vi "Host_SetParameters.vi"() -> ()   [LabVIEW 2017]
doc: "Allows manual modification of run parameters while Host__Main.vi is running.\nParameters include: distance and time thresholds for run, direction, throttle, minimum and maximum health check values, loop periods\nVI will update all values when window is closed or when \"Close Window\" button is pressed\n\nVI is automatically called on starting Host__Main.vi in order to set loop periods in Master__Main.vi.\nIf vi is not executed before running Master__Main.vi, the cRIO will not run and will return an error."
uses:
  Master/TypeDef_RunParameters.ctl
  Master/TypeDef_LoopPeriods.ctl
  Master/DAQ/Master_DataControl.ctl
  Master/DAQ/TypeDef_cRIOData.ctl
  Master/IMU/TypeDef_IMUData.ctl
  Master/CAN/TypeDef_BMSData.ctl
  Master/CAN/TypeDef_BMS_Status.ctl
  Master/CAN/MotorController/fixedMotorData.ctl
  Master/CAN/MotorController/MotorStatus.ctl
  Globals/Host_RUNPARAMETERS.vi
panel:
  in  "Disconnect Timeout (ms)":u32=30000
  in  "driveMode":enum16{"velocityMode", "torqueMode", ""}(ring)
  in  "Service Parameters":T1={"Distance Threshold (ft)"=10000.0, "Time Threshold (s)"=10000.0, "Target (I16)"=2} {"Target (I16)" min=0 max=5 step=1}
  in  "Full Run Parameters":T1={"Distance Threshold (ft)"=2300.0, "Time Threshold (s)"=12.57, "Target (I16)"=2} {"Target (I16)" min=0 max=5 step=1}
  in  "Reinitialize Network Stream":bool
  in  "Reinitialize CAN":bool
  in  "Reset Navigation":bool
  in  "Nav Period (ms)":u32=10
  in  "Set Acceleration Offset":bool
  in  "Set Min/Max Values":string[][](table)=[["22", "29.2", "V"], ["-1", "30", "A"], ["0", "0", "V"], ["-1", "30", "psig"], ["33", "149", "°F"], ["33", "248", "°F"], ["0", "1.9", "in"], ["0", "1.9", "in"], ["250", "3000", "psig"], ["-1", "15", "psig"], ["-1", "35", "psig"], ["-2.5", "20", "psig"], ["-2", "1.5", "g"], ["0", "16", "psia"], ["-40", "185", "°F"], ["33", "175", "°F"], ["10", "91", "%"], ["0", "4.1", "V"]]
  in  "CAN Period (ms)":i64=90
  in  "IMU Period (ms)":u32=5
  in  "DAQ Period (ms)":u32=100
  in  "Control Period (ms)":i64=10
  in  "Process Stop Button":bool
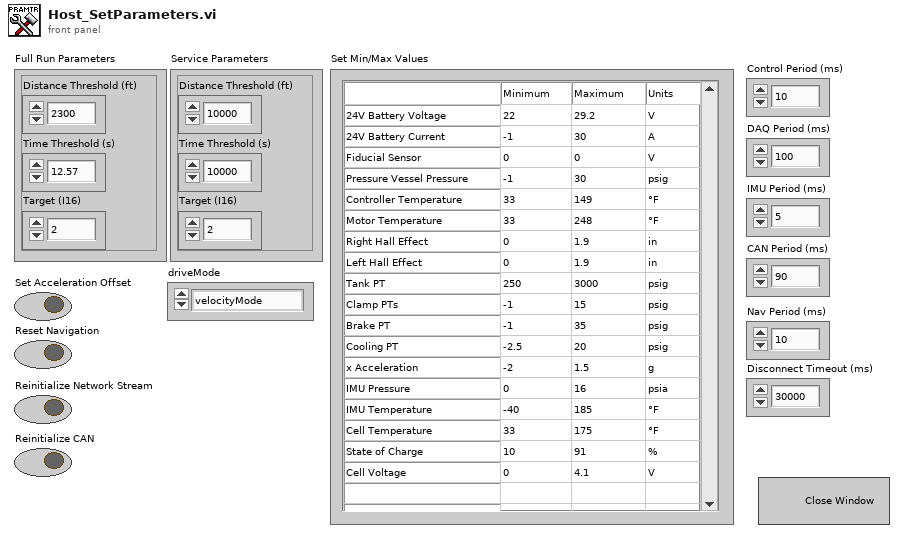
[diagram p1: front panel]
types:
  T1 = typedef "TypeDef_RunParameters.ctl" = cluster{"Distance Threshold (ft)":dbl, "Time Threshold (s)":dbl, "Target (I16)":i16}
  T2 = typedef "TypeDef_LoopPeriods.ctl" = cluster{"Control Period":i64, "DAQ Period":u32, "IMU Period":u32, "CAN Period":i64, "Nav Period":u32}
  T3 = typedef "Master_DataControl.ctl" = cluster{"cRIO Data":T4, "IMU Data":T5, "BMS Data":T6, "Motor Data":T8}
  T4 = typedef "TypeDef_cRIOData.ctl" = cluster{"Time (ms)":dbl, "24V Battery (V)":dbl, "LowV Current (A)":dbl, "Fiducial Sensor (V)":dbl, "PV Pressure (psig)":dbl, "Flow Sensor (V)":dbl, "Temp Fairing (F)":dbl, "Temp Reservoir (F)":dbl, "HallEffect Right (in)":dbl, "HallEffect Left (in)":dbl, "PT Tank (psig)":dbl, "PT Clamp Right (psig)":dbl, "PT Clamp Left (psig)":dbl, "PT Brake (psig)":dbl, "PT Cooling (psig)":dbl, "Displacement (ft)":dbl, "Velocity (ft/s)":dbl}
  T5 = typedef "TypeDef_IMUData.ctl" = cluster{"x acceleration (g)":dbl, "Pressure (psia)":dbl, "Temperature (F)":dbl}
  T6 = typedef "TypeDef_BMSData.ctl" = cluster{"Max Cell Voltage (V)":dbl, "Max Cell ID":dbl, "Min Cell Voltage (V)":dbl, "Min Cell ID":dbl, "State of Charge (%)":dbl, "Average Voltage (V)":dbl, "Voltage Delta (V)":dbl, "Pack Current (A)":dbl, "Pack Voltage (V)":dbl, "Max Resistance (Ohm)":dbl, "Min Resistance (Ohm)":dbl, "Average Resistance (Ohm)":dbl, "Delta Resistance (Ohm)":dbl, "Highest Temperature(F)":dbl, "BmsStatus":T7}
  T7 = typedef "TypeDef_BMS_Status.ctl" = cluster{"isFault":bool, "isolationMonitoring":bool}
  T8 = typedef "fixedMotorData.ctl" = cluster{"Velo (RPM)":dbl, "MotorTemp(F)":dbl, "CtrlTemp(F)":dbl, "DcLinkVolt(V)":dbl, "ErrorCode":dbl, "motorStatus":T9, "isAlive":bool, "motorControllerState":u16}
  T9 = typedef "MotorStatus.ctl" = cluster{"isReady":bool, "isOn":bool, "isOperEn":bool, "isFault":bool, "isVoltEn":bool, "targetReached":bool, "isWarning":bool}
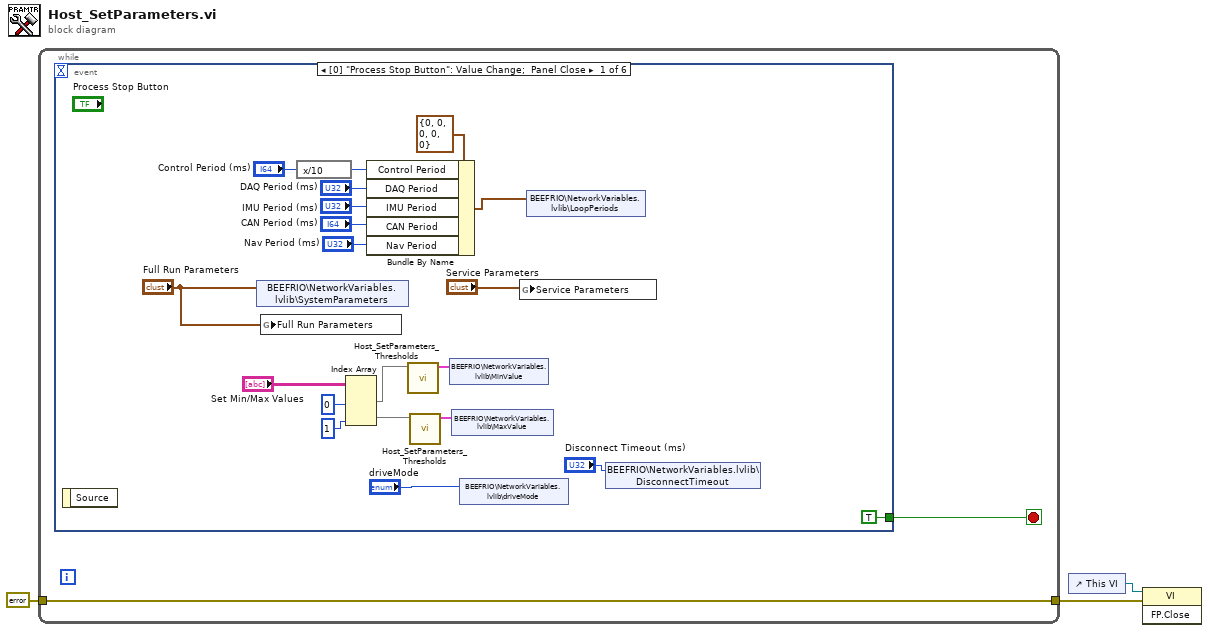
[diagram p0: block diagram]
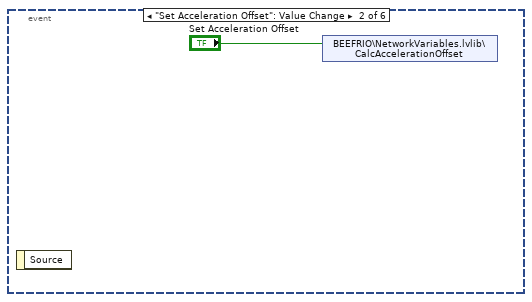
[diagram p2: hidden frame]
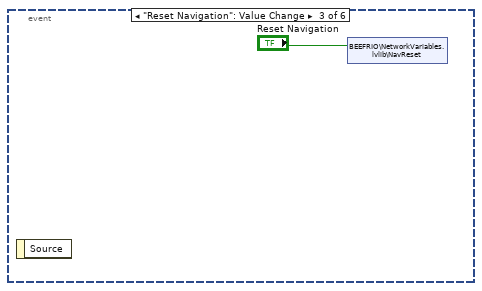
[diagram p3: hidden frame]
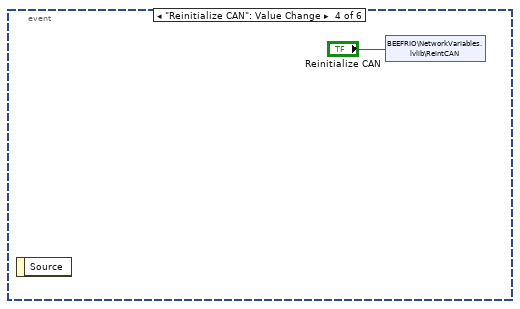
[diagram p4: hidden frame]
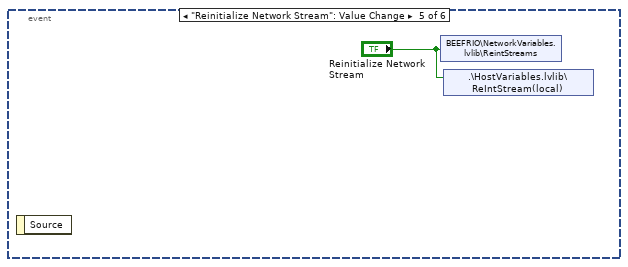
[diagram p5: hidden frame]
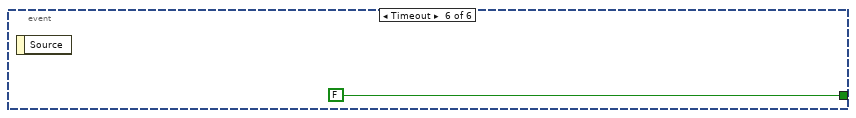
[diagram p6: hidden frame]
diagram:
  n1 = while {
    tunnel: errorcluster {"status"=FALSE, "code"=0, "source"=""} ("error IO") -> [w4]
    tunnel: [w4] -> w1
    stop <- w5 stop-if-true
    n2 = event shown="[0] \"Process Stop Button\": Value Change;  Panel Close" {
      selector: _ -> [_ _ _ _ _ _]
      dyn-events: _ -> [_ _ _ _ _ _]
      timeout: _ -> [_ _ _ _ _ _]
      tunnel: [TRUE _ _ _ _ FALSE] -> w5
      event "Process Stop Button": Value Change; Panel Close {
        n3 = event-data() -> ()  [unwired: 1 in, 1 out]
        n4 = shared-variable "BEEFRIO\\NetworkVariables.lvlib\\SystemParameters"("Full Run Parameters") -> ()  [unwired: 1 in, 1 out]
        n5 = global write "Host_RUNPARAMETERS.vi" "Full Run Parameters"("Full Run Parameters") -> ()
        n6 = expression code="x/10"("Control Period (ms)") -> (w21:i64)
        n7 = Index Array(array="Set Min/Max Values", index (col) #1=0 ("disabled index (col)"), index (col) #2=1 ("index (col)")) -> (element #1=w24:string[], element #2=w11:string[])  [unwired: 2 in]
        n8 = Bundle By Name(cluster=T2 {"Control Period"=0, "DAQ Period"=0, "IMU Period"=0, "CAN Period"=0, "Nav Period"=0} ("input cluster"), "Control Period"=w21, "DAQ Period"="DAQ Period (ms)", "IMU Period"="IMU Period (ms)", "CAN Period"="CAN Period (ms)", "Nav Period"="Nav Period (ms)") -> (w22:T2)
        n9 = call "Host_SetParameters_Thresholds.vi"("Set Min/Max Values"=w24) -> ("Data"=w10:T3)  [unwired: 10 in]
        n10 = call "Host_SetParameters_Thresholds.vi"("Set Min/Max Values"=w11) -> ("Data"=w9:T3)  [unwired: 10 in]
        n11 = shared-variable "BEEFRIO\\NetworkVariables.lvlib\\MinValue"(w10) -> ()  [unwired: 1 in, 1 out]
        n12 = shared-variable "BEEFRIO\\NetworkVariables.lvlib\\MaxValue"(w9) -> ()  [unwired: 1 in, 1 out]
        n13 = shared-variable "BEEFRIO\\NetworkVariables.lvlib\\driveMode"("driveMode") -> ()  [unwired: 1 in, 1 out]
        n14 = global write "Host_RUNPARAMETERS.vi" "Service Parameters"("Service Parameters") -> ()
        n15 = shared-variable "BEEFRIO\\NetworkVariables.lvlib\\LoopPeriods"(w22) -> ()  [unwired: 1 in, 1 out]
        n16 = shared-variable "BEEFRIO\\NetworkVariables.lvlib\\DisconnectTimeout"("Disconnect Timeout (ms)") -> ()  [unwired: 1 in, 1 out]
      }
      event "Set Acceleration Offset": Value Change {
        n17 = event-data() -> ()  [unwired: 1 in, 1 out]
        n18 = shared-variable "BEEFRIO\\NetworkVariables.lvlib\\CalcAccelerationOffset"("Set Acceleration Offset") -> ()  [unwired: 1 in, 1 out]
      }
      event "Reset Navigation": Value Change {
        n19 = event-data() -> ()  [unwired: 1 in, 1 out]
        n20 = shared-variable "BEEFRIO\\NetworkVariables.lvlib\\NavReset"("Reset Navigation") -> ()  [unwired: 1 in, 1 out]
      }
      event "Reinitialize CAN": Value Change {
        n21 = event-data() -> ()  [unwired: 1 in, 1 out]
        n22 = shared-variable "BEEFRIO\\NetworkVariables.lvlib\\ReintCAN"("Reinitialize CAN") -> ()  [unwired: 1 in, 1 out]
      }
      event "Reinitialize Network Stream": Value Change {
        n23 = event-data() -> ()  [unwired: 1 in, 1 out]
        n24 = shared-variable "BEEFRIO\\NetworkVariables.lvlib\\ReintStreams"("Reinitialize Network Stream") -> ()  [unwired: 1 in, 1 out]
        n25 = shared-variable ".\\HostVariables.lvlib\\ReIntStream(local)"("Reinitialize Network Stream") -> ()  [unwired: 1 in, 1 out]
      }
      event Timeout {
        n26 = event-data() -> ()  [unwired: 1 in, 1 out]
      }
    }
  }
  n27 = control-ref of="This VI"() -> (w3:refnum<vi>)
  n28 = invoke class="VI" method="FP.Close"(reference=w3, error in=w1) -> ()  [unwired: 1 in, 3 out]
